vi "Search.vi"(6 "Index in":i32=-1, 7 "Composite Object":refnum<class "CConfig Object.lvclass">, 8 "error in (no error)":errorcluster, 11 "Find Query in":refnum<class "All Type Query.lvclass">) -> (0 "error out":errorcluster, 2 "empty?":bool, 3 "Find Query out":refnum<class "All Type Query.lvclass">, 5 "Composite Object":refnum<class "CConfig Object.lvclass">)   [LabVIEW 2013, in "All Type Query.lvclass"]
doc: "Copyright 2018, Carya Automatisering, Wiebe Walstra."
uses:
  All Type Query.lvclass
  CConfig Object.lvclass
  Data.ctl
  All Type Query.lvclass/All Type Query.ctl
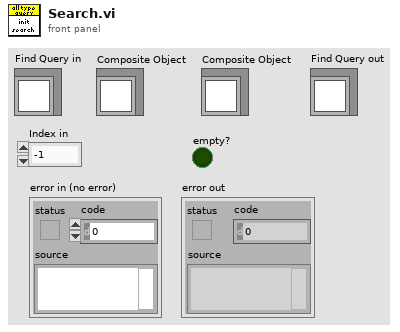
[diagram p1: front panel]
types:
  T1 = typedef "CConfig Object.lvclass/Data.ctl" = enum16{"pre", "name", "middle", "value", "post", "newline", "persistant", "tagged", "type"}
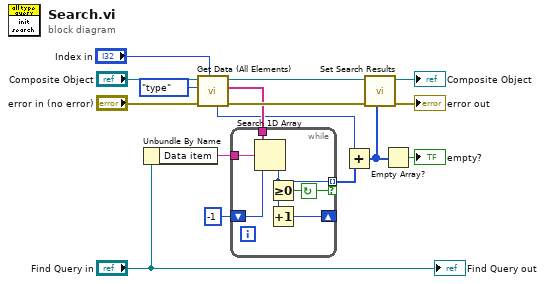
[diagram p0: block diagram]
diagram:
  n1 = Unbundle By Name("Find Query in") -> ("Data item"=w2:string)
  n2 = call "Get Data (All Elements).vi"("Start index [0]"="Index in", "error in (no error)"="error in (no error)", "Data [name]"=Data."type", "Composite Object in"="Composite Object") -> ("error out"=w8:errorcluster, "Data"=w4:string[], "Composite Object out"=w3:refnum<class "CConfig Object.lvclass">, "First part"=w1:i32)  [unwired: 4 in]
  n3 = while {
    tunnel: w4 -> [w21]
    shift-right: [w20] -> _
    shift-left: -1 ("index of element") -> [w22]
    tunnel: [w18] -> w7 mode=indexing if=w17
    tunnel: w2 -> [w19]
    stop <- w17 continue-if-true
    n4 = Search 1D Array(1D array=w21, element=w19, start index (0)=w22) -> (index of element=w18:i32)
    n5 = Greater Or Equal To 0?(x=w18) -> (x >= 0?=w17:bool)
    n6 = Increment(x=w18) -> (x+1=w20:i32)
  }
  n7 = Add(x=w1, y=w7) -> (x+y=w10:i32[])
  n8 = call-dynamic "Set Search Results.vi"("Search results"=w10, "error in (no error)"=w8, "Composite Object in"=w3) -> ("error out"=→"error out":errorcluster, "Composite Object out"=→"Composite Object":refnum<class "CConfig Object.lvclass">)  [unwired: 7 in]
  n9 = Empty Array?(array=w10) -> (empty?=→"empty?":bool)
  "Find Query out" <- "Find Query in"
